vi "HamburgerMenu.Overlay.vi"(8 "error in (no error)":errorcluster, 10 "Show / Hide (F=Hide)":bool, 11 "Owner VI Ref":refnum<vi>) -> (0 "error out":errorcluster, 3 "Owner VI Ref dup":refnum<vi>)   [LabVIEW 2014]
uses:
  Projects/NI-Days-Touch-UI/source/reuse/ApplicationControl/TypeDefs/WorkspaceReference--Enum.ctl
panel:
  out "Screen Boolean":bool
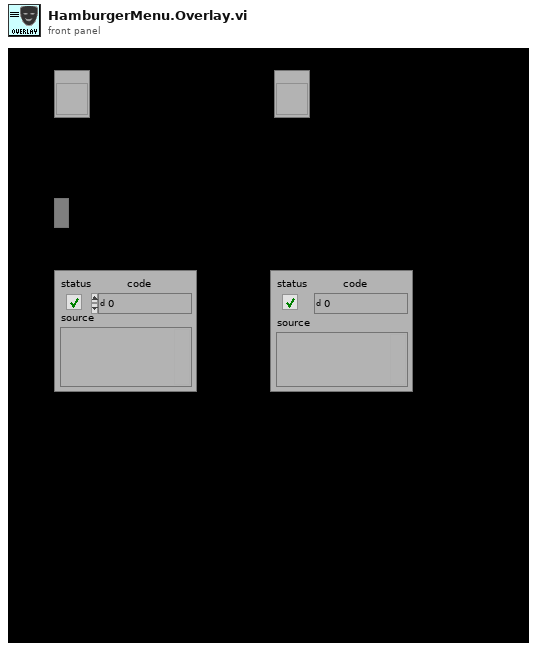
[diagram p1: front panel]
types:
  T1 = enum32{"Invalid", "Standard", "Closed", "Hidden", "Minimized", "Maximized"}
  T2 = typedef "WorkspaceReference--Enum.ctl" = enum16{"Parent Panel", "Primary Workspace", "Secondary Workspace"}
  T3 = typedef "LVRectTypeDef.ctl" = cluster{"Left":i16, "Top":i16, "Right":i16, "Bottom":i16}
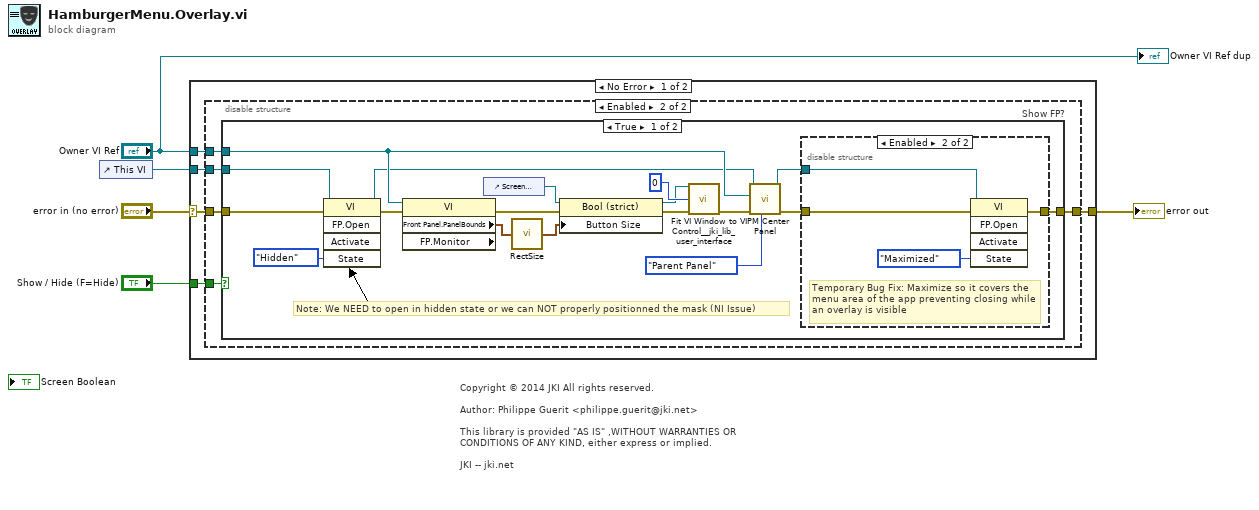
[diagram p0: block diagram]
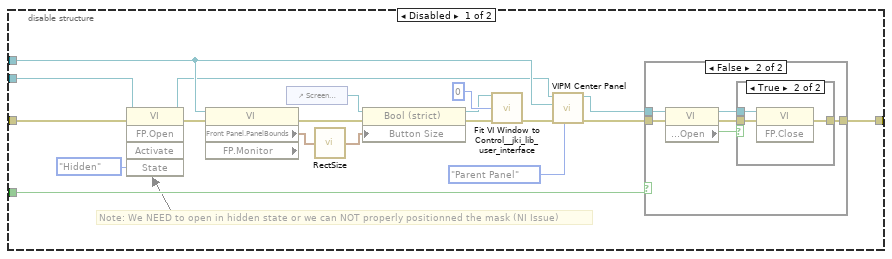
[diagram p2: hidden frame]
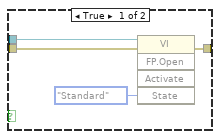
[diagram p3: hidden frame]
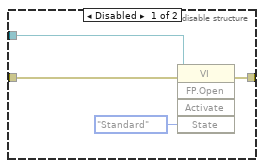
[diagram p5: hidden frame]
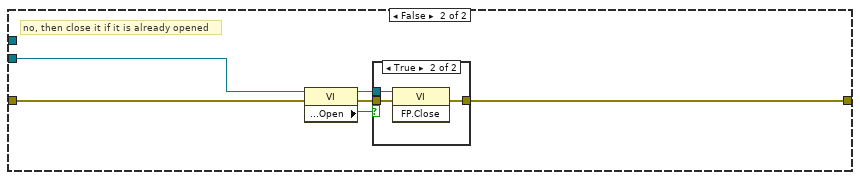
[diagram p6: hidden frame]
diagram:
  # "Copyright © 2014 JKI All rights reserved.\n\nAuthor: Philippe Guerit <philippe.guerit@jki.net>\n\nThis library is provided \"AS IS\" ,WITHOUT WARRANTIES OR \nCONDITIONS OF ANY KIND, either express or implied.\n\nJKI -- jki.net"
  n1 = control-ref of="This VI"() -> (w1:refnum<vi>)
  n2 = case shown="No Error" "error in (no error)" {
    selector: "error in (no error)" -> [w7 w85]
    tunnel: "Owner VI Ref" -> [w8 _]
    tunnel: [w10 w85] -> w5
    tunnel: "Show / Hide (F=Hide)" -> [w9 _]
    tunnel: w1 -> [w6 _]
    frame No Error {
      n3 = disable-structure shown="Enabled" {
        disable-tunnel: [w22 w48] -> w10
        disable-tunnel: w9 -> [w21 w45]
        disable-tunnel: w8 -> [w18 w47]
        disable-tunnel: w7 -> [w14 w46]
        disable-tunnel: w6 -> [w11 w44]
        frame Disabled {
          # "Note: We NEED to open in hidden state or we can NOT properly positionned the mask (NI Issue)"
          n4 = invoke class="VI" method="FP.Open"(reference=w11, error in=w14, "State"=T1."Hidden") -> (reference out=w12:refnum<vi>, error out=w13:errorcluster)  [unwired: 2 in, 3 out]
          n5 = property class="VI" props=["Front Panel.PanelBounds", "FP.Monitor"](reference=w18, error in=w13) -> (error out=w27:errorcluster, "Front Panel.PanelBounds"=w29:T3)  [unwired: 2 out]
          n6 = control-ref of="Screen Boolean"() -> (w25:refnum<vi>)
          n7 = call <vilib>:"RectSize.vi"("rect"=w29) -> ("point"=w28:cluster{"x":i16, "y":i16})
          n8 = property class="Bool (strict)"(reference=w25, error in=w27, "Button Size"=w28) -> (reference out=w24:refnum<vi>, error out=w19:errorcluster)
          n9 = call <vilib>:"Fit VI Window to Control__jki_lib_user_interface.vi"("Control Ref"=w24, "border spacing"=0, "error in (no error)"=w19) -> ("error out"=w16:errorcluster)  [unwired: 11 in, 1 out]
          n10 = call "VIPM Center Panel.vi"("Reference (workspace)"=WorkspaceReference--Enum."Parent Panel", "error in (no error)"=w16, "Parent VI Refnum"=w18, "Current VI Refnum"=w12) -> ("error out"=w23:errorcluster, "Current VI Refnum out"=w17:refnum<vi>)  [unwired: 6 in]
          n11 = case shown="False" w21 {
            tunnel: w17 -> [w33 w35]
            tunnel: w23 -> [w32 w36]
            tunnel: [w31 w34] -> w22
            frame True {
              n12 = invoke class="VI" method="FP.Open"(reference=w33, error in=w32, "State"=T1."Standard") -> (error out=w31:errorcluster)  [unwired: 2 in, 4 out]
            }
            frame False {
              n13 = property class="VI"(reference=w35, error in=w36) -> (reference out=w38:refnum<vi>, error out=w39:errorcluster, "Front Panel.Open"=w37:bool)
              n14 = case shown="True" w37 {
                tunnel: [w40 w43] -> w34
                tunnel: w39 -> [w40 w42]
                tunnel: w38 -> [_ w41]
                frame False {
                }
                frame True {
                  n15 = invoke class="VI" method="FP.Close"(reference=w41, error in=w42) -> (error out=w43:errorcluster)  [unwired: 1 in, 2 out]
                }
              }
            }
          }
        }
        frame Enabled {
          n16 = case "Show FP?" shown="True" w45 {
            tunnel: [w59 w80] -> w48
            tunnel: w47 -> [w56 _]
            tunnel: w46 -> [w52 w76]
            tunnel: w44 -> [w49 w75]
            frame True {
              # "Note: We NEED to open in hidden state or we can NOT properly positionned the mask (NI Issue)"
              n17 = invoke class="VI" method="FP.Open"(reference=w49, error in=w52, "State"=T1."Hidden") -> (reference out=w50:refnum<vi>, error out=w51:errorcluster)  [unwired: 2 in, 3 out]
              n18 = property class="VI" props=["Front Panel.PanelBounds", "FP.Monitor"](reference=w56, error in=w51) -> (error out=w64:errorcluster, "Front Panel.PanelBounds"=w66:T3)  [unwired: 2 out]
              n19 = control-ref of="Screen Boolean"() -> (w62:refnum<vi>)
              n20 = call <vilib>:"RectSize.vi"("rect"=w66) -> ("point"=w65:cluster{"x":i16, "y":i16})
              n21 = property class="Bool (strict)"(reference=w62, error in=w64, "Button Size"=w65) -> (reference out=w61:refnum<vi>, error out=w57:errorcluster)
              n22 = call <vilib>:"Fit VI Window to Control__jki_lib_user_interface.vi"("Control Ref"=w61, "border spacing"=0, "error in (no error)"=w57) -> ("error out"=w54:errorcluster)  [unwired: 11 in, 1 out]
              n23 = call "VIPM Center Panel.vi"("Reference (workspace)"=WorkspaceReference--Enum."Parent Panel", "error in (no error)"=w54, "Parent VI Refnum"=w56, "Current VI Refnum"=w50) -> ("error out"=w60:errorcluster, "Current VI Refnum out"=w55:refnum<vi>)  [unwired: 6 in]
              n24 = disable-structure shown="Enabled" {
                disable-tunnel: w60 -> [w70 w74]
                disable-tunnel: [w69 w73] -> w59
                disable-tunnel: w55 -> [w68 w72]
                frame Disabled {
                  n25 = invoke class="VI" method="FP.Open"(reference=w68, error in=w70, "State"=T1."Standard") -> (error out=w69:errorcluster)  [unwired: 2 in, 4 out]
                }
                frame Enabled {
                  # "Temporary Bug Fix: Maximize so it covers the menu area of the app preventing closing while an overlay is visible"
                  n26 = invoke class="VI" method="FP.Open"(reference=w72, error in=w74, "State"=T1."Maximized") -> (error out=w73:errorcluster)  [unwired: 2 in, 4 out]
                }
              }
            }
            frame False {
              # "no, then close it if it is already opened"
              n27 = property class="VI"(reference=w75, error in=w76) -> (reference out=w78:refnum<vi>, error out=w79:errorcluster, "Front Panel.Open"=w77:bool)
              n28 = case shown="True" w77 {
                tunnel: [w81 w84] -> w80
                tunnel: w79 -> [w81 w83]
                tunnel: w78 -> [_ w82]
                frame False {
                }
                frame True {
                  n29 = invoke class="VI" method="FP.Close"(reference=w82, error in=w83) -> (error out=w84:errorcluster)  [unwired: 1 in, 2 out]
                }
              }
            }
          }
        }
      }
    }
    frame Error {
    }
  }
  "error out" <- w5
  "Owner VI Ref dup" <- "Owner VI Ref"
